vi "tirf-initialize-handle.vi"() -> (3 "handle":i32)   [LabVIEW 2014]
uses:
  TIRF-Lock_Upgrade/TIRF-Lock/program files/Mad City Labs/TIRF-Lock/TIRF-Lock.dll
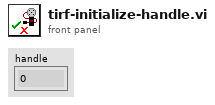
[diagram p1: front panel]
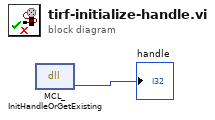
[diagram p0: block diagram]
diagram:
  n1 = dll-call lib="C:/Users/Bakir/Desktop/TIRF-Lock_Upgrade/TIRF-Lock/program files/Mad City Labs/TIRF-Lock/TIRF-Lock.dll" fn="MCL_InitHandleOrGetExisting"() -> ("handle"=→"handle":i32)  [unwired: 3 in, 2 out]
